vi "JLX.vi"() -> ()   [LabVIEW 2020]
panel:
  in  "JLX":dbl
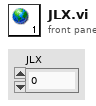
[diagram p1: front panel]
diagram:
